vi "Close.vi"(8 "Error In":errorcluster {"code" format="%.0x"}, 11 "Cards In":cluster{"Session":u32, "Card number":u32}[](array[cluster])) -> (0 "Error Out":errorcluster {"code" format="%.0x"})   [LabVIEW 2012, in "Virtual-PGA.lvlib"]
doc: "This VI closes communication with the switch and allows other applications to begin communicating with the switch unit."
uses:
  Virtual-PGA.lvlib
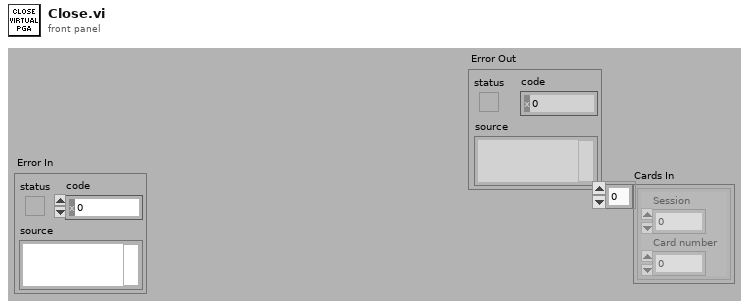
[diagram p1: front panel]
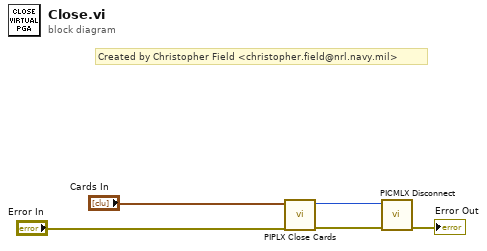
[diagram p0: block diagram]
diagram:
  # "Created by Christopher Field <christopher.field@nrl.navy.mil>"
  n1 = call <instrlib>:"PIPLX Close Cards.vi"("Input handles"="Cards In", "error in"="Error In") -> ("Session"=w2:u32, "error out"=w1:errorcluster)  [unwired: 7 in]
  n2 = call <instrlib>:"PICMLX Disconnect.vi"("error in"=w1, "Session"=w2) -> ("error out"=→"Error Out":errorcluster)  [unwired: 9 in]
